vi "Drawing Rebuild.vi"() -> ()   [LabVIEW 2021]
uses:
  <vilib>/BLE/type_def/address_type.ctl
  <vilib>/BLE/type_def/connection_status_bundle.ctl
  <vilib>/BLE/ble_functions/ble_write_by_service_characteristic_uint8array.vi
  <vilib>/Utility/inputDevices.llb/mouseAcquire.vi
panel:
  out "Connected":bool
  out "Device Name":string
  out "Handle table":string[][](array[string])
  out "Connection Status":T1={"MAC Address"="", "cnx handle"=0, "cnx flags"=0, "Address Type"=125, "Connection Interval (ms)"=125, "Timeout(ms)"=125, "Latency"=0, "bonding handle"=0} {"Address Type" items=["Public", "Random"]}
  out "Scanning":bool
  in  "Continue":bool
  in  "MAC Address":string
  in  "Address Type":T2=1 items=["Public", "Random"]
  in  "COM Bluegiga in":refnum<visa-resource-name>="COM13"
  out "Devices":string[][](array[string])
  out "BLED112 Dongle Info":string
  in  "Clear Drawing":bool
  out "Current Mouse Coordinates":T3
  out "Drawing":cluster{i32[], i32[]}[](graph)
  out "Mouse Status":cluster{"Clicked?":bool}
  in  "Emergency Stop":bool
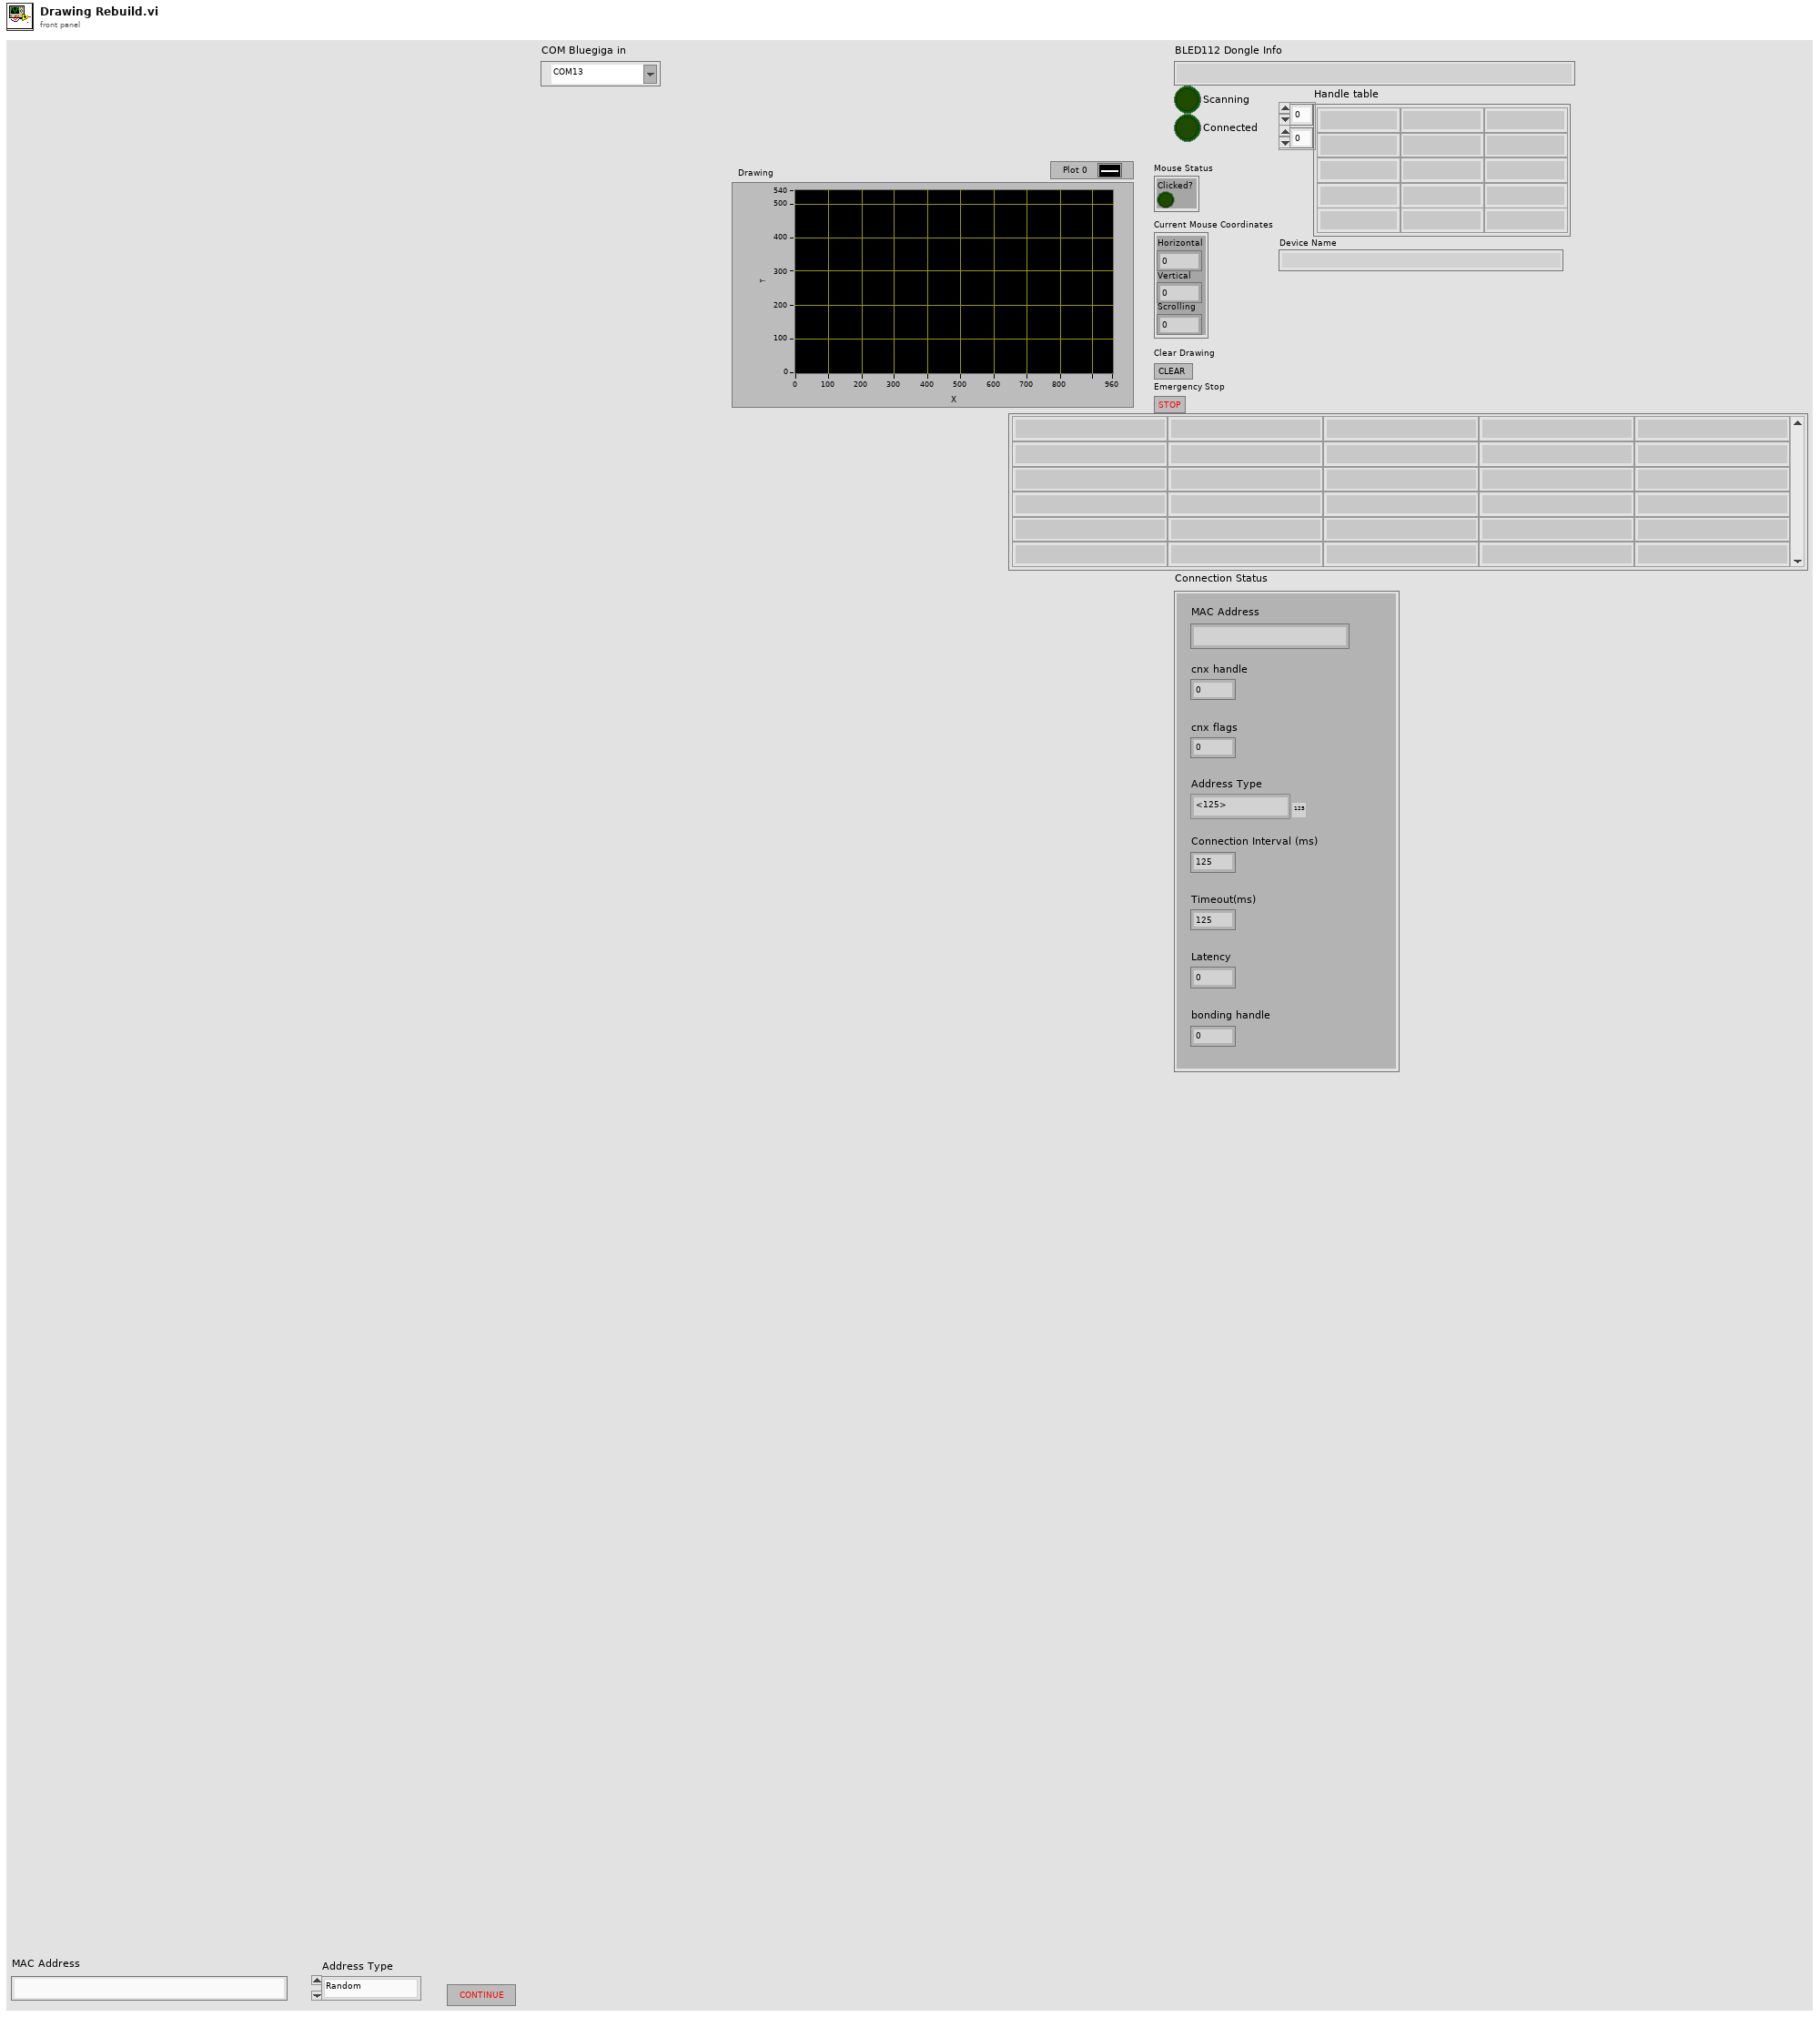
[diagram p1: front panel]
types:
  T1 = typedef "connection_status_bundle.ctl" = cluster{"MAC Address":string, "cnx handle":u8, "cnx flags":u8, "Address Type":T2, "Connection Interval (ms)":u16, "Timeout(ms)":u16, "Latency":u16, "bonding handle":u8}
  T2 = typedef "address_type.ctl" = u8
  T3 = cluster{"Horizontal":i32, "Vertical":i32, "Scrolling":i32}
  T4 = cluster{"Horizontal Array":i32[], "Vertical Array":i32[]}
  T5 = cluster{"Horizontal Array":i32[], "Vertical Array":i32[]}[]
  T6 = cluster{"button 1":bool, "button 2":bool, "button 3":bool, "button 4":bool}
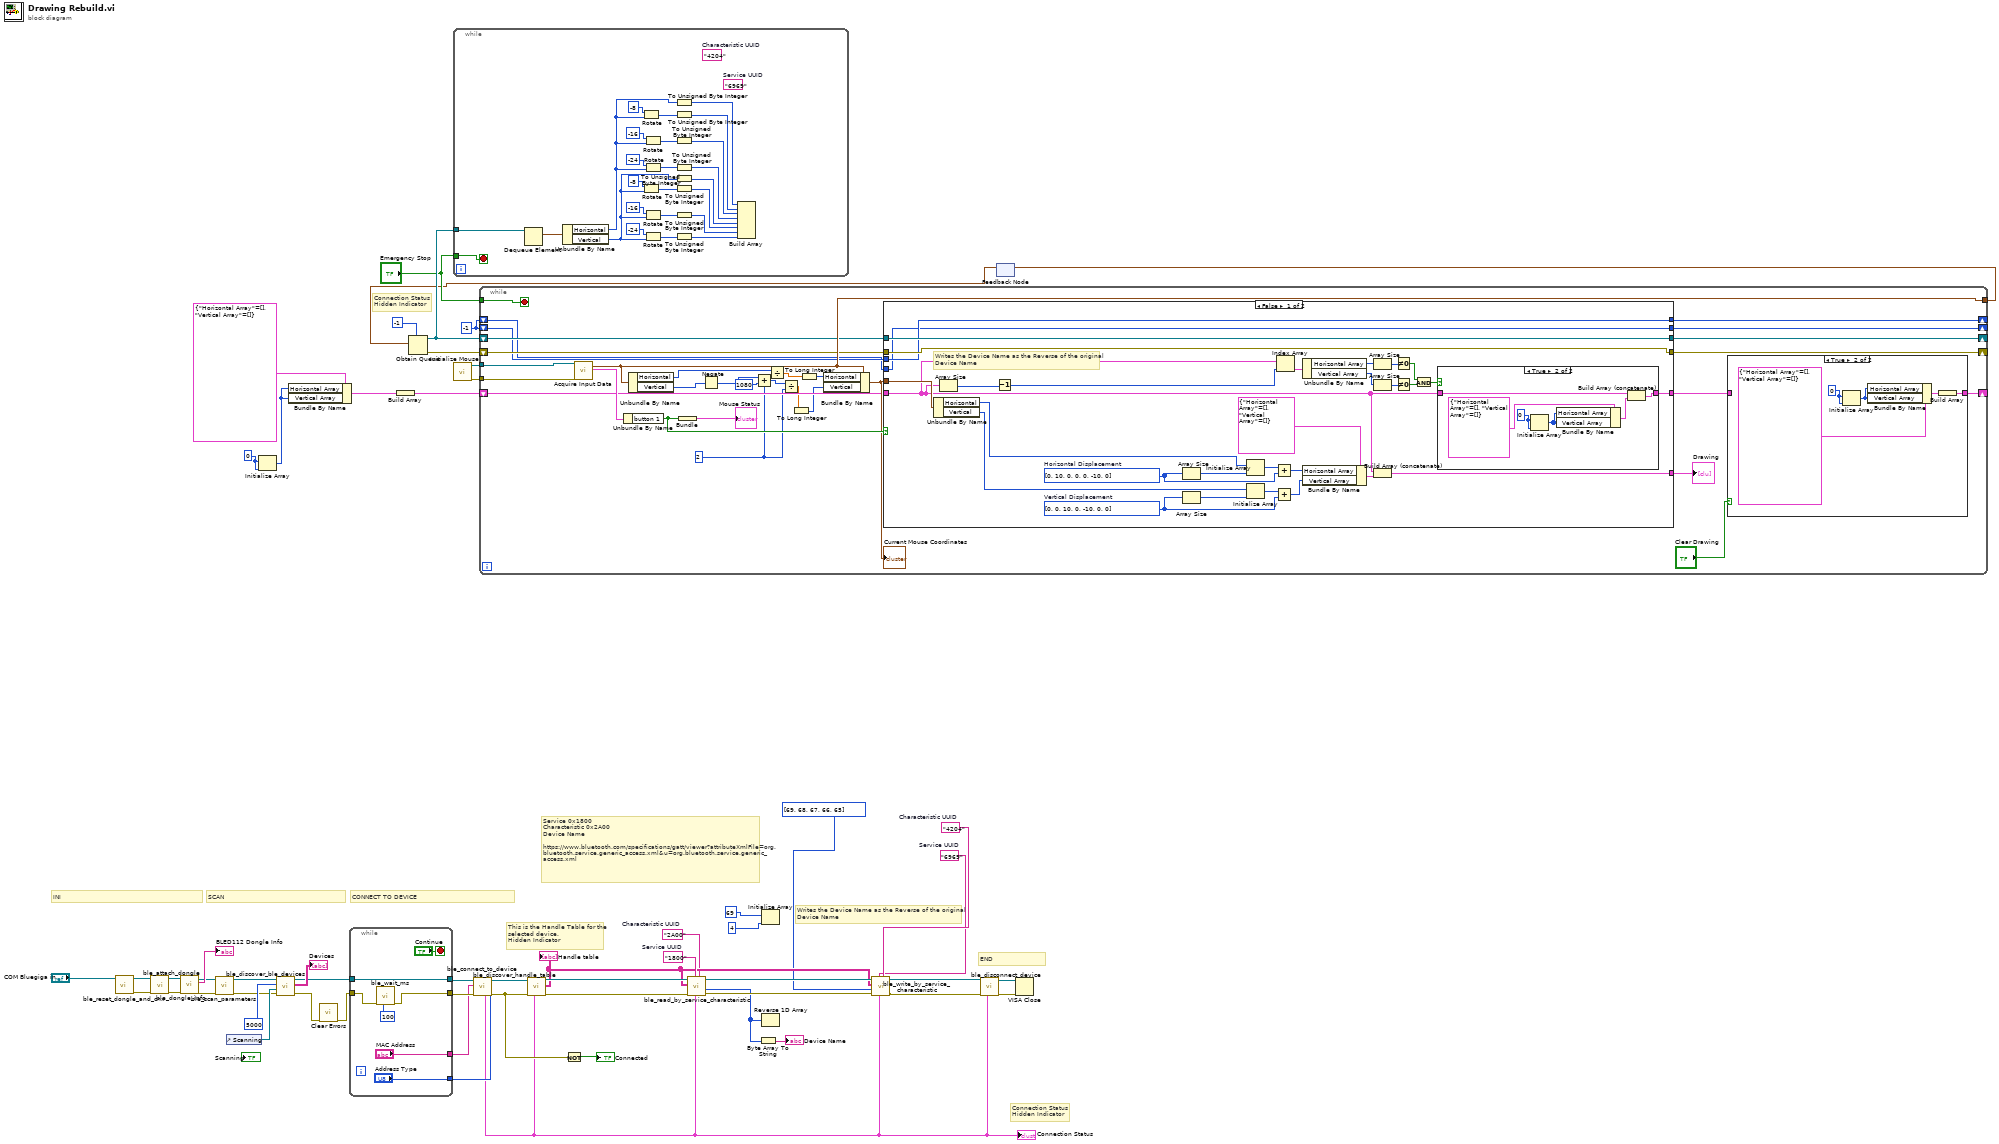
[diagram p0: block diagram]
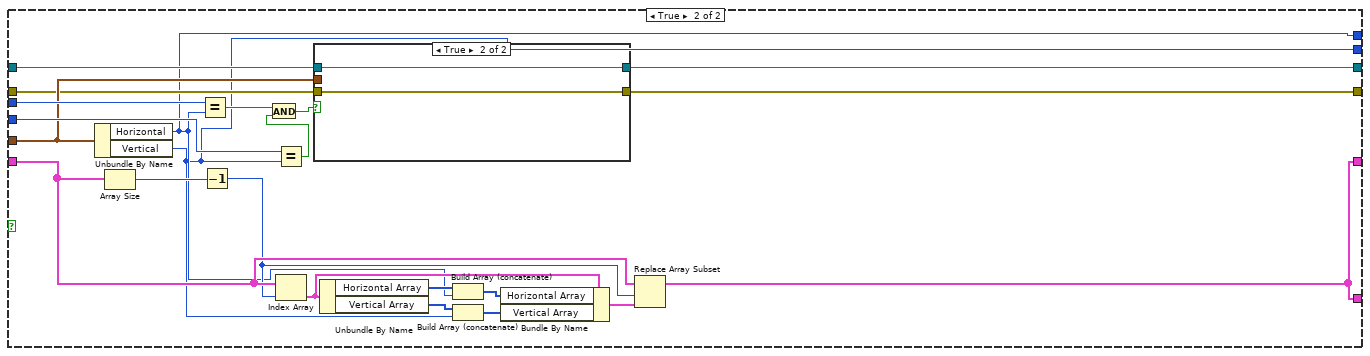
[diagram p4: hidden frame]
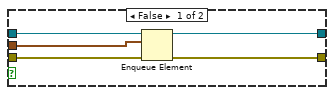
[diagram p5: hidden frame]
diagram:
  w4 = "6969"  # Service UUID
  w5 = "4204"  # Characteristic UUID
  w6 = "2A00"  # Characteristic UUID
  w11 = "1800"  # Service UUID
  w43 = -1
  w52 = 0
  # "Writes the Device Name as the Reverse of the original\nDevice Name"
  # "Connection Status\nHidden Indicator"
  # "Service 0x1800\nCharacteristic 0x2A00\nDevice Name\n\nhttps://www.bluetooth.com/specifications/gatt/viewer?attributeXmlFile=org.bluetooth.service.generic_access.xml&u=org.bluetooth.service.generic_access.xml"
  # "This is the Handle Table for the\nselected device. \nHidden Indicator"
  # "CONNECT TO DEVICE"
  # "SCAN"
  # "END"
  # "INI"
  # "Connection Status\nHidden Indicator"
  n1 = call <vilib>:"ble_reset_dongle_and_cnx.vi"("COM Bluegiga in"="COM Bluegiga in") -> ("error out"=w26:errorcluster, "COM Bluegiga out"=w24:refnum<visa-resource-name>)  [unwired: 9 in]
  n2 = call <vilib>:"ble_attach_dongle.vi"("error in (no error)"=w26, "COM Bluegiga in"=w24) -> ("error out"=w28:errorcluster, "COM Bluegiga out"=w27:refnum<visa-resource-name>)  [unwired: 8 in]
  n3 = call <vilib>:"ble_dongle_info.vi"("error in (no error)"=w28, "COM Bluegiga in"=w27) -> ("error out"=w34:errorcluster, "info"=→"BLED112 Dongle Info":string, "COM Bluegiga out"=w35:refnum<visa-resource-name>)  [unwired: 7 in]
  n4 = call <vilib>:"ble_scan_parameters.vi"("error in (no error)"=w34, "COM Bluegiga in"=w35) -> ("error out"=w32:errorcluster, "COM Bluegiga out"=w33:refnum<visa-resource-name>)  [unwired: 7 in, 1 out]
  n5 = control-ref of="Scanning"() -> (w38:refnum<vi>)
  n6 = Initialize Array(w52, w52) -> (w50:i32[])
  n7 = call <vilib>:"ble_discover_ble_devices.vi"("error in (no error)"=w32, "LED ref"=w38, "Scan Duration (10000ms)"=u32 5000, "COM Bluegiga in"=w33) -> ("error out"=w22:errorcluster, "Devices"=→"Devices":string[][], "COM Bluegiga out"=w39:refnum<visa-resource-name>)  [unwired: 5 in]
  n8 = Bundle By Name(cluster=T4 {"Horizontal Array"=[], "Vertical Array"=[]}, "Horizontal Array"=w50, "Vertical Array"=w50) -> (w53:T4)
  n9 = call <vilib>:"Clear Errors.vi"("error in (no error)"=w22) -> ("error out"=w21:errorcluster)  [unwired: 5 in, 1 out]
  n10 = while {
    tunnel: w21 -> [w62]
    tunnel: [w61] -> w37
    tunnel: w39 -> [w61]
    tunnel: [w60] -> w36
    tunnel: ["MAC Address"] -> w29
    tunnel: ["Address Type"] -> w20
    stop <- "Continue" stop-if-true
    n11 = call <vilib>:"ble_wait_ms.vi"("milliseconds to wait (100)"=u32 100, "error in (no error)"=w62) -> ("error out"=w60:errorcluster)  [unwired: 9 in]
  }
  n12 = Build Array(w53) -> (w51:T5)
  n13 = call <vilib>:"Initialize Mouse.vi"() -> ("error out"=w55:errorcluster, "device ID"=w56:refnum<k1>)  [unwired: 10 in]
  n14 = call <vilib>:"ble_connect_to_device.vi"("Address Type"=w20, "error in (no error)"=w36, "MAC Address"=w29, "COM Bluegiga in"=w37) -> ("error out"=w15:errorcluster, "COM Bluegiga out"=w23:refnum<visa-resource-name>, "Connection Status"=w12:T1)  [unwired: 5 in]
  "Connection Status" <- w12
  n15 = call <vilib>:"ble_discover_handle_table.vi"("Connection Status"=w12, "error in (no error)"=w15, "COM Bluegiga in"=w23) -> ("error out"=w19:errorcluster, "Handle table"=w10:string[][], "COM Bluegiga out"=w18:refnum<visa-resource-name>)  [unwired: 6 in]
  "Handle table" <- w10
  n16 = Not(x=w15) -> (.not. x?=→"Connected":bool)
  n17 = call <vilib>:"ble_read_by_service_characteristic.vi"("Characteristic UUID"=w6, "Connection Status"=w12, "Service UUID"=w11, "error in (no error)"=w19, "Handle table"=w10, "COM Bluegiga in"=w18) -> ("error out"=w13:errorcluster, "attribute value"=w7:u8[], "COM Bluegiga out"=w14:refnum<visa-resource-name>)  [unwired: 2 in, 1 out]
  n18 = Byte Array To String(unsigned byte array=w7) -> (string=→"Device Name":string)
  n19 = Initialize Array(u8 69, 4) -> ()  [unwired: 1 out]
  n20 = Reverse 1D Array(array=w7) -> ()  [unwired: 1 out]
  n21 = call-poly <vilib>:"ble_write_by_service_characteristic.vi"("Characteristic UUID"=w5, "Connection Status"=w12, "Service UUID"=w4, "error in (no error)"=w13, "data"=u8[] [69, 68, 67, 66, 65], "Handle table"=w10, "COM Bluegiga in"=w14) -> ("error out"=w9:errorcluster, "COM Bluegiga out"=w8:refnum<visa-resource-name>)  [unwired: 3 in]
  n22 = call <vilib>:"ble_disconnect_device.vi"("Connection Status"=w12, "error in (no error)"=w9, "COM Bluegiga in"=w8) -> ("error out"=w30:errorcluster, "COM Bluegiga out"=w31:refnum<visa-resource-name>)  [unwired: 7 in]
  n23 = feedback #1() -> (w44:T3)  [unwired: 1 in]
  n24 = Obtain Queue(max queue size (-1, unlimited)=-1, element data type=w44) -> (queue out=w47:refnum<queue>, error out=w48:errorcluster)  [unwired: 3 in, 1 out]
  n25 = while {
    tunnel: w47 -> [w68]
    tunnel: "Emergency Stop" -> [w64]
    stop <- w64 stop-if-true
    (unwired) "6969"  # Service UUID
    (unwired) "4204"  # Characteristic UUID
    n26 = Dequeue Element(queue=w68) -> (element=w67:T3)  [unwired: 2 in, 3 out]
    n27 = Unbundle By Name(w67) -> ("Horizontal"=w66:i32, "Vertical"=w65:i32)
    n28 = Rotate(1:w66, 2:-8) -> (0:w79:i32)
    n29 = Rotate(1:w65, 2:-8) -> (0:w82:i32)
    n30 = Rotate(1:w66, 2:-16) -> (0:w80:i32)
    n31 = Rotate(1:w66, 2:-24) -> (0:w81:i32)
    n32 = Rotate(1:w65, 2:-16) -> (0:w83:i32)
    n33 = Rotate(1:w65, 2:-24) -> (0:w84:i32)
    n34 = To Unsigned Byte Integer(number=w66) -> (unsigned 8bit integer=w75:u8)
    n35 = To Unsigned Byte Integer(number=w79) -> (unsigned 8bit integer=w78:u8)
    n36 = To Unsigned Byte Integer(number=w80) -> (unsigned 8bit integer=w77:u8)
    n37 = To Unsigned Byte Integer(number=w81) -> (unsigned 8bit integer=w76:u8)
    n38 = To Unsigned Byte Integer(number=w65) -> (unsigned 8bit integer=w85:u8)
    n39 = To Unsigned Byte Integer(number=w82) -> (unsigned 8bit integer=w86:u8)
    n40 = To Unsigned Byte Integer(number=w83) -> (unsigned 8bit integer=w87:u8)
    n41 = To Unsigned Byte Integer(number=w84) -> (unsigned 8bit integer=w88:u8)
    n42 = Build Array(w75, w78, w77, w76, w85, w86, w87, w88) -> ()  [unwired: 1 out]
  }
  n43 = while {
    tunnel: w56 -> [w119]
    tunnel: w55 -> [w118]
    shift-right: [w108] -> _
    shift-left: w51 -> [w112]
    tunnel: [w105] -> w45
    shift-right: [w101] -> _
    shift-left: w47 -> [w104]
    shift-right: [w102] -> _
    shift-left: w48 -> [w103]
    tunnel: "Emergency Stop" -> [w100]
    shift-right: [w97] -> _
    shift-left: w43 -> [w99]
    shift-right: [w96] -> _
    shift-left: w43 -> [w98]
    stop <- w100 stop-if-true
    w91 = 2
    n44 = call-poly <vilib>:"Acquire Input Data.vi"("device ID"=w119, "error in (no error)"=w118) -> ("axis info"=w105:T3, "button info"=w117:T6)  [unwired: 14 in, 2 out]
    n45 = Unbundle By Name(w117) -> ("button 1"=w114:bool)
    n46 = Unbundle By Name(w105) -> ("Horizontal"=w92:i32, "Vertical"=w116:i32)
    n47 = Bundle("button 1"=w114) -> (→"Mouse Status":cluster{"button 1":bool})  [unwired: 1 in]
    n48 = Negate(x=w116) -> (-x=w107:i32)
    n49 = Add(x=w107, y=1080) -> (x+y=w93:i32)
    n50 = Divide(x=w92, y=w91) -> (x/y=w89:dbl)
    n51 = Divide(x=w93, y=w91) -> (x/y=w95:dbl)
    n52 = To Long Integer(number=w95) -> (32bit integer=w94:i32)
    n53 = To Long Integer(number=w89) -> (32bit integer=w90:i32)
    n54 = Bundle By Name(cluster=w105, "Horizontal"=w90, "Vertical"=w94) -> (w113:T3)
    "Current Mouse Coordinates" <- w113
    n55 = case shown="False" w114 {
      tunnel: w112 -> [w142 w178]
      tunnel: w113 -> [w144 w170]
      tunnel: [w145 w175] -> w109
      tunnel: [w140 w175] -> w111
      tunnel: w104 -> [w129 w166]
      tunnel: w103 -> [w128 w169]
      tunnel: [w128 w167] -> w102
      tunnel: [w129 w168] -> w101
      tunnel: w99 -> [w127 w173]
      tunnel: w98 -> [w126 w172]
      tunnel: [w127 w164] -> w97
      tunnel: [w126 w163] -> w96
      frame False {
        w134 = i32[] [0, 0, 10, 0, -10, 0, 0]  # Vertical Displacement
        w136 = i32[] [0, 10, 0, 0, 0, -10, 0]  # Horizontal Displacement
        # "Writes the Device Name as the Reverse of the original\nDevice Name"
        n56 = Unbundle By Name(w144) -> ("Horizontal"=w131:i32, "Vertical"=w130:i32)
        n57 = Array Size(array=w142) -> (size(s)=w153:i32)
        n58 = Decrement(x=w153) -> (x-1=w155:i32)
        n59 = Array Size(array=w136) -> (size(s)=w139:i32)
        n60 = Array Size(array=w134) -> (size(s)=w138:i32)
        n61 = Initialize Array(w131, w139) -> (w137:i32[])
        n62 = Initialize Array(w130, w138) -> (w135:i32[])
        n63 = Add(x=w137, y=w136) -> (x+y=w132:i32[])
        n64 = Add(x=w135, y=w134) -> (x+y=w133:i32[])
        n65 = Index Array(array=w142, index=w155) -> (element=w154:T4)
        n66 = Unbundle By Name(w154) -> ("Horizontal Array"=w152:i32[], "Vertical Array"=w151:i32[])
        n67 = Bundle By Name(cluster=T4 {"Horizontal Array"=[], "Vertical Array"=[]}, "Horizontal Array"=w132, "Vertical Array"=w133) -> (w141:T4)
        n68 = Array Size(array=w152) -> (size(s)=w150:i32)
        n69 = Array Size(array=w151) -> (size(s)=w149:i32)
        n70 = Build Array (concatenate)(w142, w141) -> (w140:T5)
        n71 = Not Equal To 0?(x=w150) -> (x != 0?=w148:bool)
        n72 = Not Equal To 0?(x=w149) -> (x != 0?=w147:bool)
        n73 = And(x=w148, y=w147) -> (x .and. y?=w146:bool)
        n74 = case shown="True" w146 {
          tunnel: w142 -> [w156 w160]
          tunnel: [w156 w157] -> w145
          frame False {
          }
          frame True {
            w161 = 0
            n75 = Initialize Array(w161, w161) -> (w162:i32[])
            n76 = Bundle By Name(cluster=T4 {"Horizontal Array"=[], "Vertical Array"=[]}, "Horizontal Array"=w162, "Vertical Array"=w162) -> (w158:T4)
            n77 = Build Array (concatenate)(w160, w158) -> (w157:T5)
          }
        }
      }
      frame True {
        n78 = Unbundle By Name(w170) -> ("Horizontal"=w164:i32, "Vertical"=w163:i32)
        n79 = Array Size(array=w178) -> (size(s)=w184:i32)
        n80 = Equal?(x=w173, y=w164) -> (x = y?=w174:bool)
        n81 = Decrement(x=w184) -> (x-1=w177:i32)
        n82 = Equal?(x=w172, y=w163) -> (x = y?=w171:bool)
        n83 = And(x=w174, y=w171) -> (x .and. y?=w165:bool)
        n84 = Index Array(array=w178, index=w177) -> (element=w181:T4)
        n85 = case shown="True" w165 {
          tunnel: w170 -> [w189 _]
          tunnel: w169 -> [w188 w190]
          tunnel: [w187 w191] -> w168
          tunnel: [w186 w190] -> w167
          tunnel: w166 -> [w185 w191]
          frame False {
            n86 = Enqueue Element(queue=w185, element=w189, error in (no error)=w188) -> (queue out=w187:refnum<queue>, error out=w186:errorcluster)  [unwired: 1 in, 1 out]
          }
          frame True {
          }
        }
        n87 = Unbundle By Name(w181) -> ("Horizontal Array"=w183:i32[], "Vertical Array"=w182:i32[])
        n88 = Build Array (concatenate)(w183, w164) -> (w180:i32[])
        n89 = Build Array (concatenate)(w182, w163) -> (w179:i32[])
        n90 = Bundle By Name(cluster=w181, "Horizontal Array"=w180, "Vertical Array"=w179) -> (w176:T4)
        n91 = Replace Array Subset(array=w178, new element=w176, index=w177) -> (w175:T5)
      }
    }
    "Drawing" <- w111
    n92 = case shown="True" "Clear Drawing" {
      tunnel: w109 -> [w120 _]
      tunnel: [w120 w121] -> w108
      frame False {
      }
      frame True {
        w123 = 0
        n93 = Initialize Array(w123, w123) -> (w125:i32[])
        n94 = Bundle By Name(cluster=T4 {"Horizontal Array"=[], "Vertical Array"=[]}, "Horizontal Array"=w125, "Vertical Array"=w125) -> (w124:T4)
        n95 = Build Array(w124) -> (w121:T5)
      }
    }
  }
  n96 = feedback-in #1(w45) -> ()
  n97 = VISA Close(VISA resource name=w31, error in (no error)=w30) -> ()  [unwired: 1 out]
